vi "sleep_horm_det.vi"(5 "Path_Sleep_list":path, 6 "Порог":dbl(slide) scale=0.0..1500.0, 7 "sec_in":dbl, 8 "df":dbl format="%.2f", 9 "FFT_in":dbl[](array[numeric]) format="%.2f", 10 "Shift_Amp_in":u16, 11 "Shift_Sleep_in":i32) -> (0 "Sleep Norm":bool, 2 "Shift_Amp_out":u16, 3 "Shift_Sleep_out":i32, 4 "PWR_OUT":T1(graph))   [LabVIEW 2013]
uses:
  <vilib>/Utility/file.llb/Write To Spreadsheet File (DBL).vi
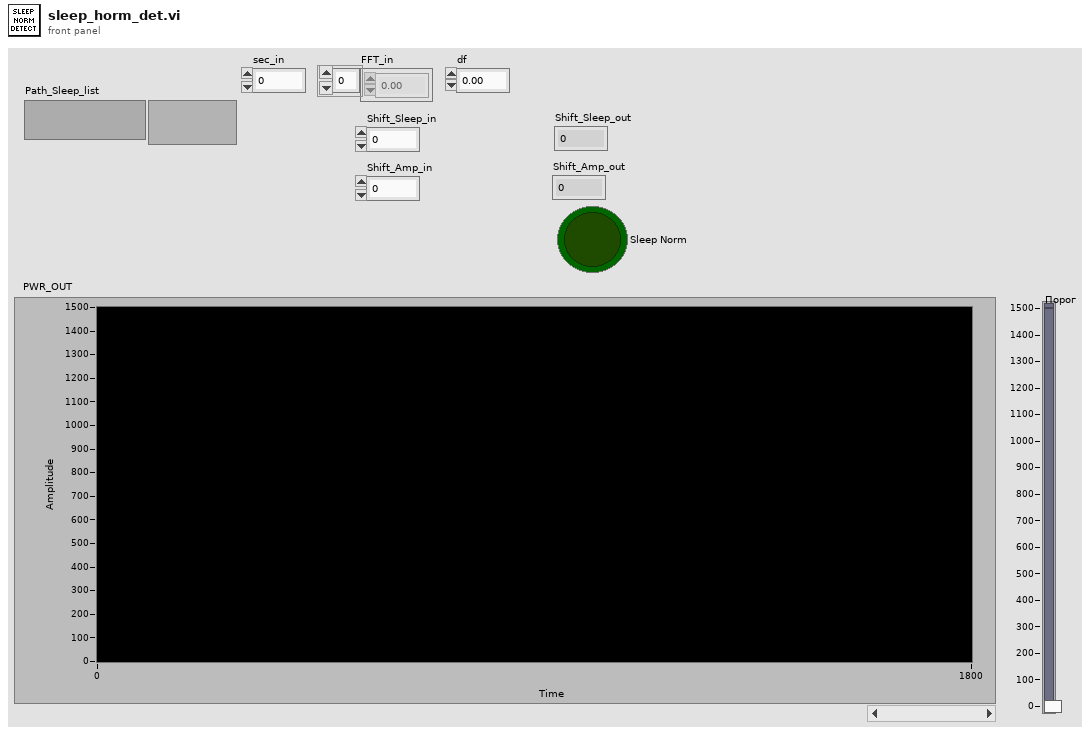
[diagram p1: front panel]
types:
  T1 = cluster{"PWR_BAND":dbl, "PWR_BAND":dbl, "PWR_BAND":dbl, "PWR_BAND":dbl, "Порог":dbl, dbl}
  T2 = cluster{"PWR_BAND":dbl, "PWR_BAND":dbl, "PWR_BAND":dbl, "PWR_BAND":dbl}
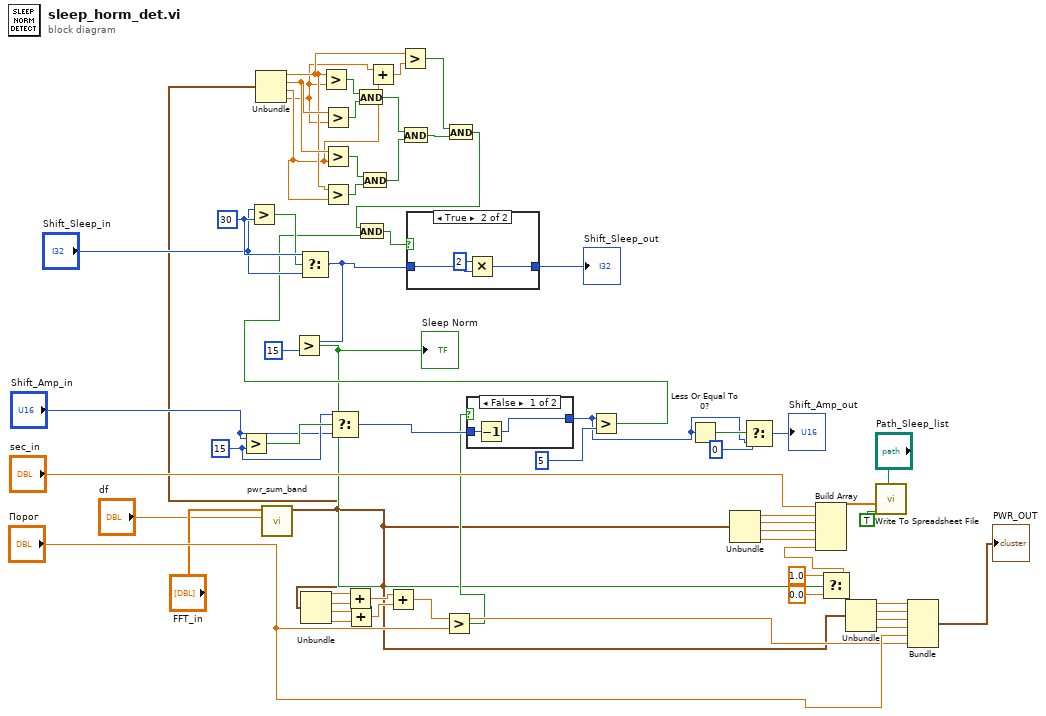
[diagram p0: block diagram]
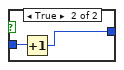
[diagram p2: hidden frame]
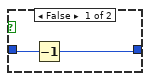
[diagram p3: hidden frame]
diagram:
  w37 = u16 15 ("y")
  w54 = 30 ("y")
  n1 = Greater?(x="Shift_Amp_in", y=w37) -> (0:w38:bool)
  n2 = Greater?(x="Shift_Sleep_in", y=w54) -> (0:w42:bool)
  n3 = call "pwr_sum_band.vi"("df"="df", "In"="FFT_in") -> ("OUT"=w1:T2)  [unwired: 9 in]
  n4 = Unbundle(w1) -> ("PWR_BAND"=w49:dbl, "PWR_BAND"=w50:dbl, "PWR_BAND"=w46:dbl, "PWR_BAND"=w45:dbl)
  n5 = Select(t=w54, s=w42, f="Shift_Sleep_in") -> (s? t:f=w43:i32)
  n6 = Greater?(x=w43, y=15) -> (0:w2:bool)
  "Sleep Norm" <- w2
  n7 = Unbundle(w1) -> ("PWR_BAND"=w26:dbl, "PWR_BAND"=w27:dbl, "PWR_BAND"=w24:dbl, "PWR_BAND"=w25:dbl)
  n8 = Greater?(x=w49, y=w45) -> (0:w58:bool)
  n9 = Greater?(x=w50, y=w45) -> (0:w57:bool)
  n10 = Greater?(x=w50, y=w46) -> (0:w59:bool)
  n11 = Greater?(x=w49, y=w46) -> (0:w60:bool)
  n12 = Select(t=w37, s=w38, f="Shift_Amp_in") -> (s? t:f=w36:u16)
  n13 = Add(x=w26, y=w27) -> (x+y=w23:dbl)
  n14 = Add(x=w24, y=w25) -> (x+y=w22:dbl)
  n15 = And(x=w58, y=w57) -> (x .and. y?=w55:bool)
  n16 = And(x=w59, y=w60) -> (x .and. y?=w56:bool)
  n17 = Add(x=w45, y=w46) -> (x+y=w44:dbl)
  n18 = Add(x=w23, y=w22) -> (x+y=w9:dbl)
  n19 = Greater?(x=w49, y=w44) -> (0:w47:bool)
  n20 = And(x=w55, y=w56) -> (x .and. y?=w48:bool)
  n21 = Greater?(x=w9, y="Порог") -> (0:w3:bool)
  n22 = And(x=w47, y=w48) -> (x .and. y?=w41:bool)
  n23 = case shown="False" w3 {
    tunnel: w36 -> [w62 w64]
    tunnel: [w61 w63] -> w11
    frame False {
      n24 = Decrement(x=w62) -> (x-1=w61:u16)
    }
    frame True {
      n25 = Increment(x=w64) -> (x+1=w63:u16)
    }
  }
  n26 = Greater?(x=w11, y=u16 5) -> (0:w13:bool)
  n27 = And(x=w41, y=w13) -> (x .and. y?=w40:bool)
  n28 = case shown="True" w40 {
    tunnel: w43 -> [w66 w69]
    tunnel: [w65 w68] -> w51
    frame False {
      n29 = Decrement(x=w66) -> (x-1=w65:i32)
    }
    frame True {
      n30 = Multiply(x=2, y=w69) -> (x*y=w68:i32)
    }
  }
  "Shift_Sleep_out" <- w51
  n31 = Less Or Equal To 0?(x=w11) -> (x <= 0?=w16:bool)
  n32 = Unbundle(w1) -> ("PWR_BAND"=w31:dbl, "PWR_BAND"=w30:dbl, "PWR_BAND"=w29:dbl, "PWR_BAND"=w28:dbl)
  n33 = Select(t=u16 0, s=w16, f=w11) -> (s? t:f=→"Shift_Amp_out":u16)
  n34 = Select(t=1.0, s=w2, f=0.0) -> (s? t:f=w32:dbl)
  n35 = Build Array("sec_in", w31, w30, w29, w28, w32) -> (w7:dbl[])
  n36 = Unbundle(w1) -> ("PWR_BAND"=w21:dbl, "PWR_BAND"=w20:dbl, "PWR_BAND"=w18:dbl, "PWR_BAND"=w17:dbl)
  n37 = call-poly <vilib>:"Write To Spreadsheet File.vi"("append to file? (new file:F)"=TRUE, "1D data"=w7, "file path (dialog if empty)"="Path_Sleep_list") -> ()  [unwired: 5 in, 1 out]
  n38 = Bundle("PWR_BAND"=w21, "PWR_BAND"=w20, "PWR_BAND"=w18, "PWR_BAND"=w17, "Порог"="Порог", w9) -> (→"PWR_OUT":T1)  [unwired: 1 in]
